vi "Vowel-Create.vi"(0 "Vowel":T1, 7 "Sampling Rate (Hz)":dbl, 9 "Npts":i32, 11 "error in (no error)":errorcluster) -> (8 "WF":dbl[](array[numeric]), 15 "error out":errorcluster)   [LabVIEW 2020]
uses:
  XControls/Waveform XControls/Vowel/Vowel.Properties.ctl
  <vilib>/Analysis/NI_AALBase.lvlib
  XControls/Waveform XControls/Vowel/Vowel.xctl
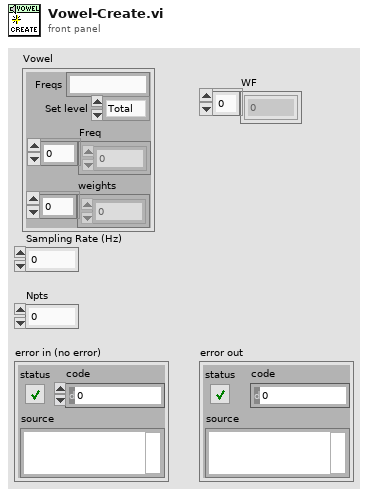
[diagram p1: front panel]
types:
  T1 = typedef "Vowel.xctl/Vowel.Properties.ctl" = cluster{"Freqs":string, "Set level":enum16{"Total", "Per component"}, "Freq":dbl[], "weights":dbl[]}
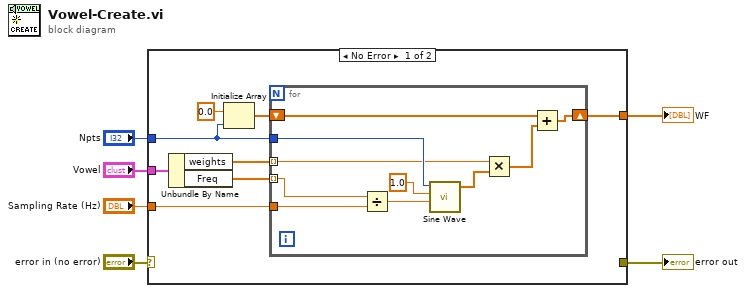
[diagram p0: block diagram]
diagram:
  n1 = case shown="No Error" "error in (no error)" {
    selector: "error in (no error)" -> [_ w25]
    tunnel: [_ w25] -> w2
    tunnel: [w7 _] -> w3
    tunnel: "Vowel" -> [w14 _]
    tunnel: "Sampling Rate (Hz)" -> [w11 _]
    tunnel: "Npts" -> [w10 _]
    frame No Error {
      n2 = Unbundle By Name(w14) -> ("weights"=w13:dbl[], "Freq"=w12:dbl[])
      n3 = Initialize Array(0.0 ("element"), w10) -> (w8:dbl[])
      n4 = for {
        tunnel: w13 -> [w18] mode=indexing
        tunnel: w12 -> [w22] mode=indexing
        tunnel: w11 -> [w21]
        tunnel: w10 -> [w20]
        shift-right: [w17] -> w7
        shift-left: w8 -> [w15]
        n5 = Divide(x=w22, y=w21) -> (x/y=w24:dbl)
        n6 = call <vilib>:"Sine Wave.vi"("samples"=w20, "amplitude"=1.0, "frequency"=w24) -> ("sine wave"=w19:dbl[])  [unwired: 2 in, 2 out]
        n7 = Multiply(x=w18, y=w19) -> (x*y=w16:dbl[])
        n8 = Add(x=w15, y=w16) -> (x+y=w17:dbl[])
      }
    }
    frame Error {
    }
  }
  "WF" <- w3
  "error out" <- w2
